vi "Pre Launch Init.vi"(11 "Motor in":refnum<class "Motor.lvclass">) -> (0 "error out":errorcluster, 3 "Motor out":refnum<class "Motor.lvclass">)   [LabVIEW 2026, in "Motor.lvlib" / "Motor.lvclass"]
doc: "<p>(<strong>Filename</strong>: <span class=\"dnl\">Actor Framework.lvlib:Actor.lvclass:Pre Launch Init.vi</span>)</p>\n<p>Defines behavior that occurs after the <a href=\"nihelplauncher://docs/csh?context=lvcore_lvcomm_af_launch_nested_actor\">Launch Nested Actor</a> method is invoked but before the actor's Actor Core method begins running.</p>\n<p>By default, this method does nothing. A descendant class may override it to define behavior.</p>"
uses:
  Motor.lvclass
  Motor.lvclass/Motor.ctl
  <vilib>/ActorFramework/Actor/Actor.lvclass
  CTI-Grove/Examples/Sourcecode/cti-drivers-lv-visa-simple/Examples/Driver/CTIPicoVISA.lvlib
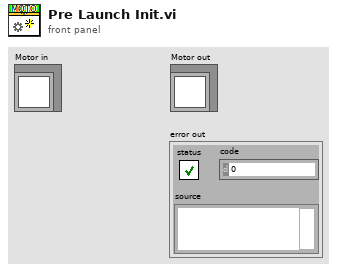
[diagram p1: front panel]
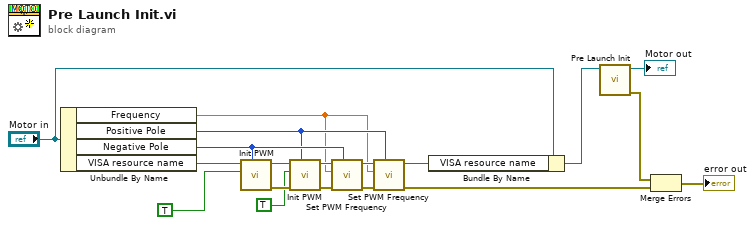
[diagram p0: block diagram]
diagram:
  n1 = Unbundle By Name("Motor in") -> ("Frequency"=w3:dbl, "Positive Pole"=w4:i32, "Negative Pole"=w5:i32, "VISA resource name"=w6:refnum<visa-resource-name>)
  n2 = call "Init PWM.vi"("GPIO"=w5, "Enable (F)"=TRUE, "VISA resource name in"=w6) -> ("error out"=w16:errorcluster, "VISA resource name"=w15:refnum<visa-resource-name>)  [unwired: 7 in]
  n3 = call "Init PWM.vi"("GPIO"=w4, "error in (no error)"=w16, "Enable (F)"=TRUE, "VISA resource name in"=w15) -> ("error out"=w7:errorcluster, "VISA resource name"=w12:refnum<visa-resource-name>)  [unwired: 6 in]
  n4 = call "Set PWM Frequency.vi"("GPIO"=w5, "error in (no error)"=w7, "Freq Hz"=w3, "VISA resource name in"=w12) -> ("error out"=w8:errorcluster, "VISA resource name"=w11:refnum<visa-resource-name>)  [unwired: 6 in]
  n5 = call "Set PWM Frequency.vi"("GPIO"=w4, "error in (no error)"=w8, "Freq Hz"=w3, "VISA resource name in"=w11) -> ("error out"=w9:errorcluster, "VISA resource name"=w1:refnum<visa-resource-name>)  [unwired: 6 in]
  n6 = Bundle By Name(cluster="Motor in", "VISA resource name"=w1) -> (w2:refnum<class "Motor.lvclass">)
  n7 = call-parent "Pre Launch Init.vi"("Actor in"=w2) -> ("error out"=w19:errorcluster, "Actor out"=→"Motor out":refnum<class "Motor.lvclass">)  [unwired: 9 in]
  n8 = Merge Errors(w19, w9) -> (→"error out":errorcluster)
